vi "write_to_text_file.vi"(8 "error in (no error)":errorcluster, 10 "Path":path, 11 "PointLinkCollection in":refnum<class "PointLinkCollection.lvclass">) -> (0 "error out":errorcluster, 3 "PointLinkCollection out":refnum<class "PointLinkCollection.lvclass">)   [LabVIEW 2010, in "PointLinkCollection.lvclass"]
uses:
  PointLinkCollection.lvclass
  PointLinkCollection.lvclass/PointLinkCollection.ctl
  <vilib>/Utility/file.llb/Write To Spreadsheet File (DBL).vi
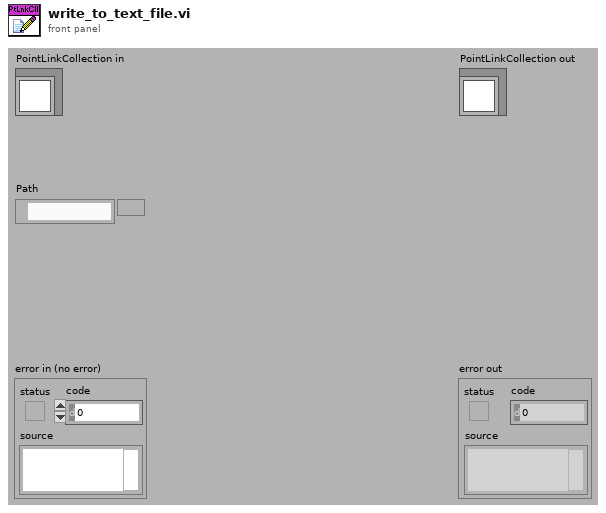
[diagram p1: front panel]
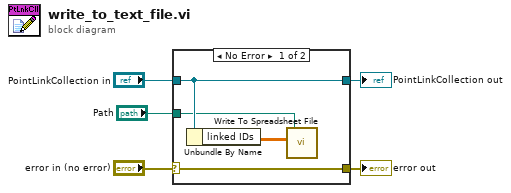
[diagram p0: block diagram]
diagram:
  n1 = case shown="No Error" "error in (no error)" {
    selector: "error in (no error)" -> [w9 w11]
    tunnel: [w9 w11] -> w4
    tunnel: [w8 w10] -> w2
    tunnel: "PointLinkCollection in" -> [w8 w10]
    tunnel: "Path" -> [w6 _]
    frame No Error {
      n2 = Unbundle By Name(w8) -> ("linked IDs"=w7:dbl[][])
      n3 = call-poly <vilib>:"Write To Spreadsheet File.vi"("2D data"=w7, "file path (dialog if empty)"=w6) -> ()  [unwired: 6 in, 1 out]
    }
    frame Error {
    }
  }
  "error out" <- w4
  "PointLinkCollection out" <- w2
